vi "Servicio Total.vi"(10 "Lista servicios in":string[][](array[string]), 11 "MulticolumnListbox in":refnum<vi>) -> (3 "Lista servicios out":string[][](array[string]))   [LabVIEW 2020, in "Manejador Turnos.lvlib"]
uses:
  Manejador Turnos.lvlib
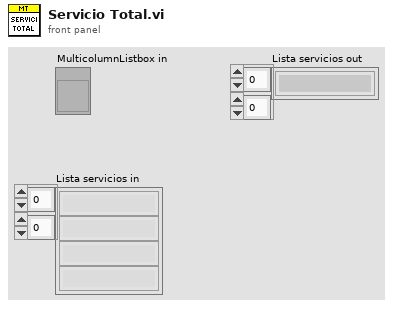
[diagram p1: front panel]
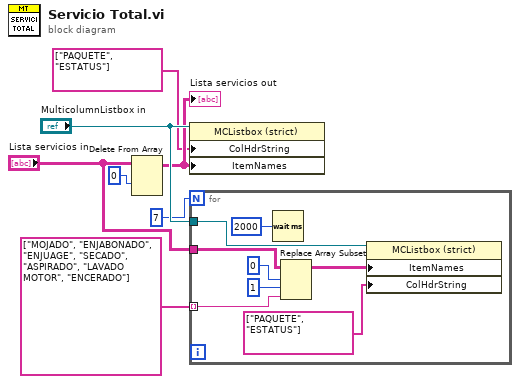
[diagram p0: block diagram]
diagram:
  n1 = Delete From Array(array="Lista servicios in", index (row)=0) -> (array with subset deleted=w5:string[][])  [unwired: 2 in, 1 out]
  "Lista servicios out" <- w5
  n2 = property on="Property Node" class="MCListbox (strict)"(reference="MulticolumnListbox in", "ColHdrString"=string[] ["PAQUETE", "ESTATUS"] ("Column Header Strings[]"), "ItemNames"=w5) -> ()  [unwired: 1 in, 2 out]
  n3 = for {
    N: 7 -> [_]
    tunnel: "Lista servicios in" -> [w15]
    tunnel: string[] ["MOJADO", "ENJABONADO", "ENJUAGE", "SECADO", "ASPIRADO", "LAVADO MOTOR", "ENCERADO"] -> [w9] mode=indexing
    tunnel: "MulticolumnListbox in" -> [w8]
    n4 = Wait (ms)(milliseconds to wait=u32 2000) -> ()  [unwired: 1 out]
    n5 = Replace Array Subset(array=w15, new element=w9, index (row)=0, index (col)=1 ("disabled index (col)")) -> (w13:string[][])
    n6 = property on="Property Node" class="MCListbox (strict)"(reference=w8, "ItemNames"=w13, "ColHdrString"=string[] ["PAQUETE", "ESTATUS"] ("Column Header Strings[]")) -> ()  [unwired: 1 in, 2 out]
  }
